vi "IMAQController.set i attribute.vi"(0 "i ref in":refnum<vi>, 2 "i attribute":T1, 5 "error in (no error)":errorcluster) -> (14 "i ref out":refnum<vi>, 19 "error out":errorcluster)   [LabVIEW 2014, in "IMAQController.lvlib"]
doc: "Sets the i attribute data of an object.\n\nLicense Agreement for this software:\n\nCopyright (C)\nGesellschaft für Schwerionenforschung, GSI\nPlanckstr. 1\n64291 Darmstadt\nGermany\n\nContact: D.Beck@gsi.de \n\nThis program is free software; you can redistribute it and/or modify it under the terms of the GNU General Public License as published by the Free Software Foundation; either version 2 of the license, or (at your option) any later version.\n\nThis program is distributed in the hope that it will be useful, but WITHOUT ANY WARRANTY; without even the implied warranty of MERCHANTABILITY or FITNESS FOR A PARTICULAR PURPOSE. See the GNU General License for more details (http://www.gnu.org).\n\nGesellschaft für Schwerionenforschung, GSI\nPlanckstr. 1, 64291 Darmstadt, Germany\nFor all questions and ideas contact: M.Richter@gsi.de, H.Brand@gsi.de or D.Beck@gsi.de.\nLast update: 17-JUN-2004"
uses:
  IMAQController.lvlib
  IMAQController.i attribute.ctl
  <vilib>/Utility/miscctls.llb/LVPoint32TypeDef.ctl
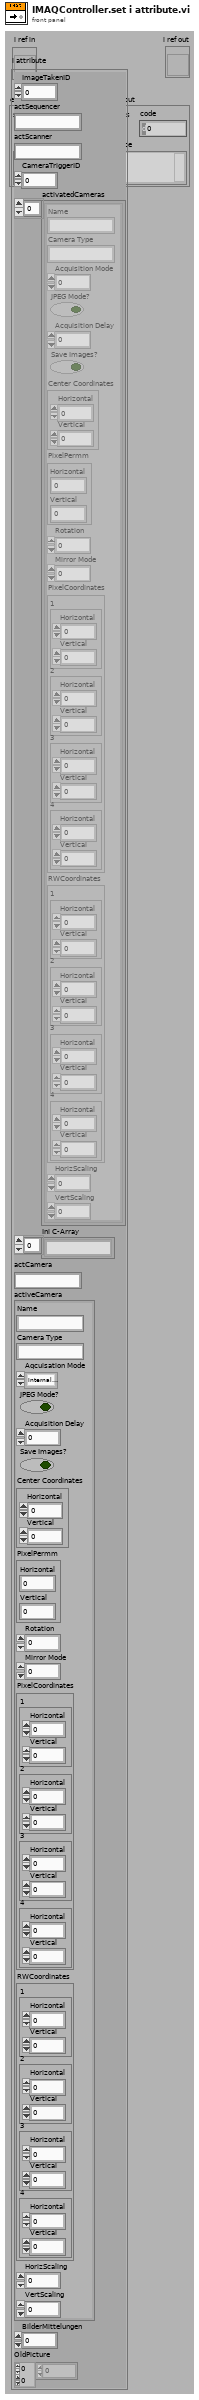
[diagram p1: front panel]
types:
  T1 = typedef "IMAQController.lvlib/IMAQController.i attribute.ctl" = cluster{"ImageTakenID":i32, "actSequencer":string, "actScanner":string, "CameraTriggerID":i32, "activatedCameras":cluster{"Name":string, "Camera Type":string, "Acquisition Mode":u32, "JPEG Mode?":bool, "Acquisition Delay":dbl, "Save Images?":bool, "Center Coordinates":T2, "PixelPermm":cluster{"Horizontal":dbl, "Vertical":dbl}, "Rotation":dbl, "Mirror Mode":u32, "PixelCoordinates":cluster{"1":cluster{"Horizontal":i32, "Vertical":i32}, "2":cluster{"Horizontal":i32, "Vertical":i32}, "3":cluster{"Horizontal":i32, "Vertical":i32}, "4":cluster{"Horizontal":i32, "Vertical":i32}}, "RWCoordinates":cluster{"1":cluster{"Horizontal":dbl, "Vertical":dbl}, "2":cluster{"Horizontal":dbl, "Vertical":dbl}, "3":cluster{"Horizontal":dbl, "Vertical":dbl}, "4":cluster{"Horizontal":dbl, "Vertical":dbl}}, "HorizScaling":dbl, "VertScaling":dbl}[], "Ini C-Array":string[], "actCamera":string, "activeCamera":cluster{"Name":string, "Camera Type":string, "Aqcuisation Mode":enum32{"Internal Trigger", "Scan", "free Running", "External Trigger"}, "JPEG Mode?":bool, "Acquisition Delay":dbl, "Save Images?":bool, "Center Coordinates":T2, "PixelPermm":cluster{"Horizontal":dbl, "Vertical":dbl}, "Rotation":dbl, "Mirror Mode":u32, "PixelCoordinates":cluster{"1":cluster{"Horizontal":i32, "Vertical":i32}, "2":cluster{"Horizontal":i32, "Vertical":i32}, "3":cluster{"Horizontal":i32, "Vertical":i32}, "4":cluster{"Horizontal":i32, "Vertical":i32}}, "RWCoordinates":cluster{"1":cluster{"Horizontal":dbl, "Vertical":dbl}, "2":cluster{"Horizontal":dbl, "Vertical":dbl}, "3":cluster{"Horizontal":dbl, "Vertical":dbl}, "4":cluster{"Horizontal":dbl, "Vertical":dbl}}, "HorizScaling":dbl, "VertScaling":dbl}, "BilderMittelungen":u8, "OldPicture":dbl[][]}
  T2 = typedef "LVPoint32TypeDef.ctl" = cluster{"Horizontal":i32, "Vertical":i32}
  T3 = enum16{"SetAttribute", "GetAttribute", "CreateAttribute", "DestroyAttribute", "DestroyAllAtributes"}
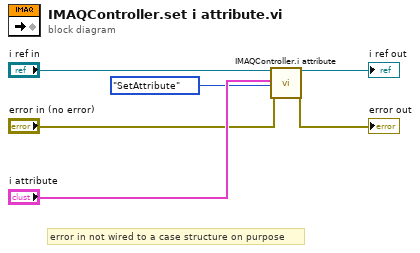
[diagram p0: block diagram]
diagram:
  # "error in not wired to a case structure on purpose"
  n1 = call "IMAQController.i attribute.vi"("VI Refnum"="i ref in", "CLASS.i attribute"="i attribute", "Action"=T3."SetAttribute", "error in (no error)"="error in (no error)") -> ("VI Refnum out"=→"i ref out":refnum<vi>, "error out"=→"error out":errorcluster)  [unwired: 13 in, 1 out]
